vi "Create Deserializer VI in Logic.vi"(0 "VI in":refnum<vi>, 5 "Term Refnum":refnum<vi>, 7 "Name Out":string, 11 "error in (no error)":errorcluster) -> (15 "error out":errorcluster)   [LabVIEW 2021, in "Migrator.lvlib"]
uses:
  Migrator.lvlib
  <vilib>/Utility/traverseref.llb/TRef TravTarget.ctl
  <vilib>/Utility/traverseref.llb/VI Scripting - Traverse.lvlib
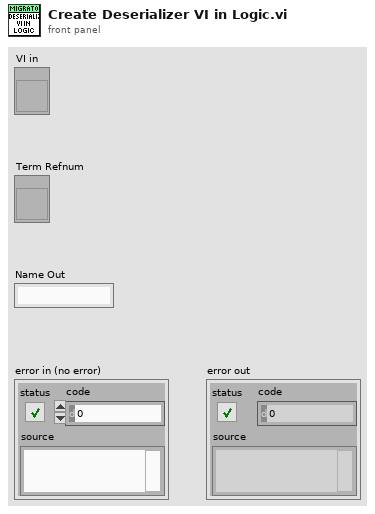
[diagram p1: front panel]
types:
  T1 = typedef "TRef TravTarget.ctl" = enum16{"FP", "BD", "Other"}
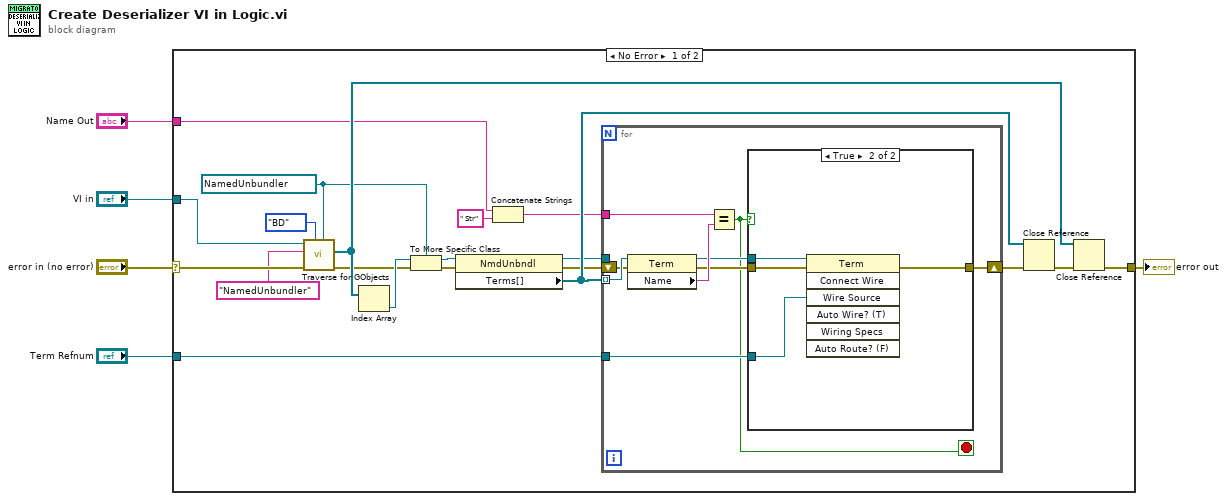
[diagram p0: block diagram]
diagram:
  n1 = case shown="No Error" "error in (no error)" {
    selector: "error in (no error)" -> [w8 w39]
    tunnel: [w23 w39] -> w5
    tunnel: "Term Refnum" -> [w20 _]
    tunnel: "Name Out" -> [w15 _]
    tunnel: "VI in" -> [w9 _]
    frame No Error {
      w11 = refnum<vi> refnum ("Other Refnum")
      n2 = call <vilib>:"Traverse for GObjects.vi"("Other Refnum"=w11, "Traverse Target"=TRef_TravTarget."BD", "error in (no error)"=w8, "Class Name"="NamedUnbundler", "VI Refnum"=w9) -> ("error out"=w10:errorcluster, "References"=w24:refnum<vi>[])  [unwired: 3 in, 2 out]
      n3 = Index Array(array=w24) -> (element=w12:refnum<vi>)  [unwired: 1 in]
      n4 = To More Specific Class(target class=w11, reference=w12, error in=w10) -> (specific class reference=w13:refnum<vi>, error out=w14:errorcluster)
      n5 = property class="NmdUnbndl"(reference=w13, error in=w14) -> (reference out=w19:refnum<vi>, error out=w18:errorcluster, "Terms[]"=w22:refnum<vi>[])
      n6 = Concatenate Strings(w15, " Str" ("string")) -> (w17:string)
      n7 = for {
        tunnel: w22 -> [w32] mode=indexing
        tunnel: w17 -> [w33]
        shift-right: [w26] -> w21
        shift-left: w18 -> [w31]
        tunnel: w19 -> [_]
        tunnel: w20 -> [w27]
        stop <- w25 stop-if-true
        n8 = property class="Term"(reference=w32, error in=w31) -> (reference out=w28:refnum<vi>, error out=w29:errorcluster, "Name"=w30:string)
        n9 = Equal?(x=w33, y=w30) -> (x = y?=w25:bool)
        n10 = case shown="True" w25 {
          tunnel: w29 -> [w34 w37]
          tunnel: w28 -> [_ w38]
          tunnel: w27 -> [_ w36]
          tunnel: [w34 w35] -> w26
          frame False {
          }
          frame True {
            n11 = invoke class="Term" method="Connect Wire"(reference=w38, error in=w37, "Wire Source"=w36) -> (error out=w35:errorcluster)  [unwired: 4 in, 6 out]
          }
        }
      }
      n12 = Close Reference(reference=w22, error in (no error)=w21) -> (error out=w23:errorcluster)
      n13 = Close Reference(reference=w24, error in (no error)=w23) -> ()  [unwired: 1 out]
    }
    frame Error {
    }
  }
  "error out" <- w5
